vi "randbool.vi"() -> (3 "Boolesch":bool)   [LabVIEW 2014]
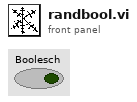
[diagram p1: front panel]
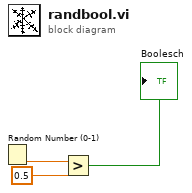
[diagram p0: block diagram]
diagram:
  n1 = Random Number (0-1)() -> (number: 0 to 1=w3:dbl)
  n2 = Greater?(x=w3, y=0.5) -> (0:→"Boolesch":bool)
